vi "FineDB_CONNECT.vi"(5 "SQL Server_Hostname":string="192.168.8.233", 6 "error in (no error)":errorcluster, 8 "password":string="CQFA8", 9 "account":string="sa", 11 "DB_name":string="CQFA8") -> (0 "error out":errorcluster, 3 "ADODB._Connection Out":refnum<k7>)   [LabVIEW 2018]
panel:
  # "Rev2.0"
  # "Output"
  # "Input"
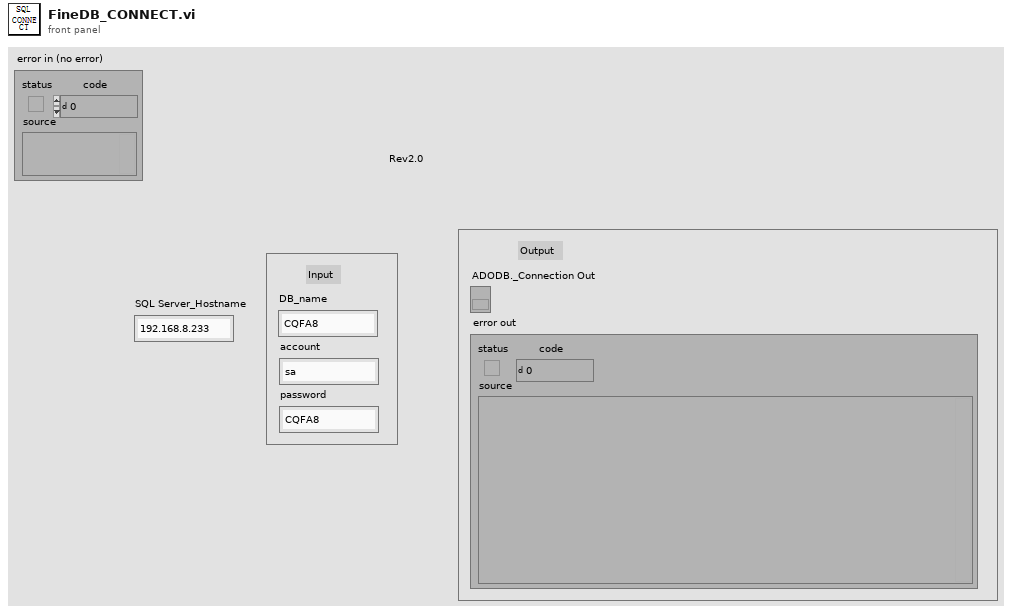
[diagram p1: front panel]
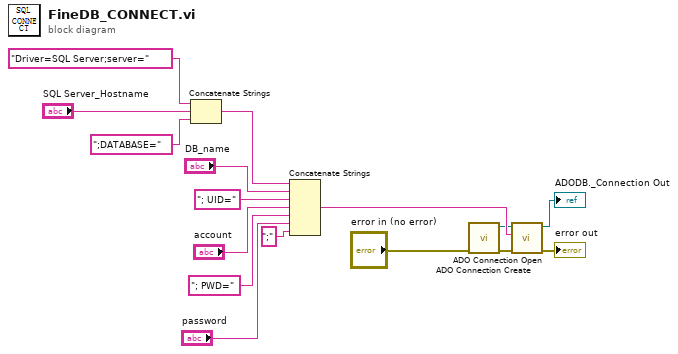
[diagram p0: block diagram]
diagram:
  n1 = Concatenate Strings("Driver=SQL Server;server=", "SQL Server_Hostname", ";DATABASE=") -> (w10:string)
  n2 = Concatenate Strings(w10, "DB_name", "; UID=" ("字符串"), "account", "; PWD=" ("字符串"), "password", ";" ("字符串")) -> (w16:string)
  n3 = call <userlib>:"ADO Connection Create.vi"("error in (no error)"="error in (no error)") -> ("error out"=w5:errorcluster, "ADODB._Connection Out"=w4:refnum<k7>)  [unwired: 9 in]
  n4 = call <userlib>:"ADO Connection Open.vi"("error in (no error)"=w5, "ConnectionString"=w16, "ADODB._Connection In"=w4) -> ("error out"=→"error out":errorcluster, "ADODB._Connection Out"=→"ADODB._Connection Out":refnum<k7>)  [unwired: 7 in]
